vi "ex_1.vi"() -> ()   [LabVIEW 2020]
uses:
  #typedef_FGV_SinusAction.ctl
panel:
  in  "dx (0,1)":dbl=0.1
  in  "stop":bool
  out "Sinus Output":dbl(graph)
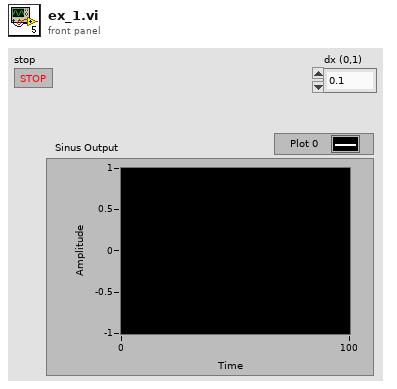
[diagram p1: front panel]
types:
  T1 = typedef "#typedef_FGV_SinusAction.ctl" = enum16{"Reset", "Increment argument"}
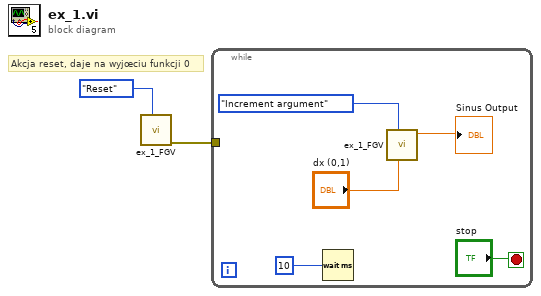
[diagram p0: block diagram]
diagram:
  # "Akcja reset, daje na wyjœciu funkcji 0"
  n1 = call "ex_1_FGV.vi"("Sinus Action  (Increment argument)"=#typedef_FGV_SinusAction."Reset") -> ("error out"=w1:errorcluster)  [unwired: 9 in, 1 out]
  n2 = while {
    tunnel: w1 -> [_]
    stop <- "stop" stop-if-true
    n3 = Wait (ms)(milliseconds to wait=u32 10) -> ()  [unwired: 1 out]
    n4 = call "ex_1_FGV.vi"("dx (0,1)"="dx (0,1)", "Sinus Action  (Increment argument)"=#typedef_FGV_SinusAction."Increment argument") -> ("Sinus output"=→"Sinus Output":dbl)  [unwired: 8 in, 1 out]
  }
